vi "Send ReplayData Msg.vi"(6 "On End Message":refnum<class "Data Msg.lvclass">, 7 "Message Priority (Normal)":T1=enum."Normal", 8 "error in (no error)":errorcluster, 9 "Caller Enqueuer":refnum<class "Message Enqueuer.lvclass">, 10 "ReplayData Msg":refnum<class "ReplayData Msg.lvclass">, 11 "Message Enqueuer":refnum<class "Message Enqueuer.lvclass">) -> (0 "error out":errorcluster, 3 "Message Enqueuer out":refnum<class "Message Enqueuer.lvclass">)   [LabVIEW 2014, in "ReplayData Msg.lvclass"]
uses:
  ReplayData Msg.lvclass
  <vilib>/ActorFramework/Message Enqueuer/Message Enqueuer.lvclass
  <vilib>/ActorFramework/Message Enqueuer/Message Priority.ctl
  Data Msg/Data Msg.lvclass
  ExperimentService/Replay Msg.lvclass
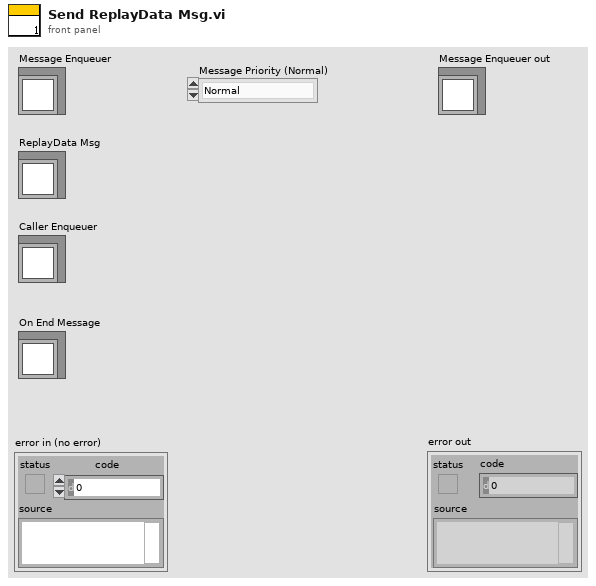
[diagram p1: front panel]
types:
  T1 = typedef "Actor Framework.lvlib/Message Enqueuer.lvclass/Message Priority.ctl" = enum16{"Low", "Normal", "High"}
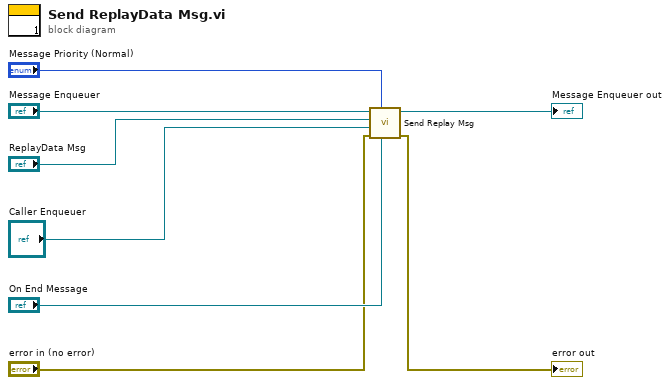
[diagram p0: block diagram]
diagram:
  n1 = call "Send Replay Msg.vi"("On End Message"="On End Message", "Message Priority (Normal)"="Message Priority (Normal)", "error in (no error)"="error in (no error)", "Caller Enqueuer"="Caller Enqueuer", "Replay Message in"="ReplayData Msg", "Message Enqueuer"="Message Enqueuer") -> ("error out"=→"error out":errorcluster, "Message Enqueuer out"=→"Message Enqueuer out":refnum<class "Message Enqueuer.lvclass">)  [unwired: 4 in]
